vi "Read.vi"(8 "error in (no error)":errorcluster, 11 "object in":refnum<class "Type-K-Thermocouple.lvclass">) -> (0 "error out":errorcluster, 2 "Data":dbl[](array[numeric]), 3 "object out":refnum<class "Type-K-Thermocouple.lvclass">)   [LabVIEW 2021, in "Type-K-Thermocouple.lvclass"]
doc: "Read converted data from modbus Reg"
uses:
  Type-K-Thermocouple.lvclass
  Modbus-Instr_class/Modbus-Instr.lvclass
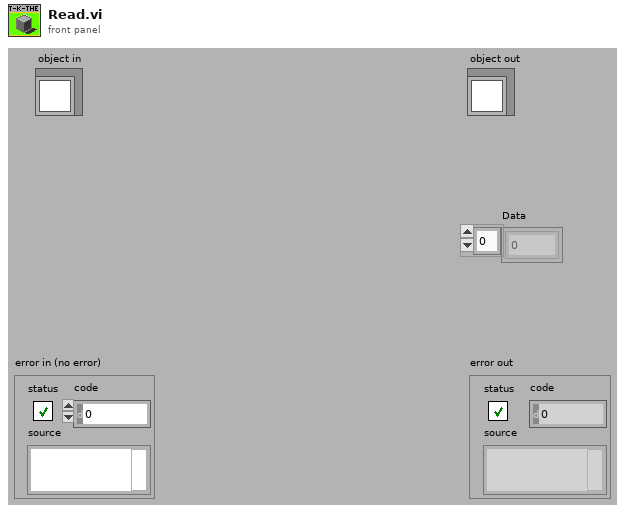
[diagram p1: front panel]
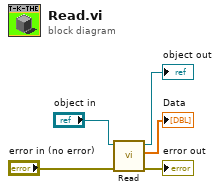
[diagram p0: block diagram]
diagram:
  n1 = call-parent "Read.vi"("error in (no error)"="error in (no error)", "object in"="object in") -> ("error out"=→"error out":errorcluster, "Data"=→"Data":dbl[], "object out"=→"object out":refnum<class "Type-K-Thermocouple.lvclass">)  [unwired: 7 in]
